vi "Override To Nominal State.vi"(11 "TEMPLATE Queue in":refnum<class "TEMPLATE Queue.lvclass">) -> (3 "TEMPLATE Queue out":refnum<class "TEMPLATE Queue.lvclass">)   [LabVIEW 2021, in "_Template.lvlib" / "Templates.lvlib" / "TEM Queue.lvlib" / "TEMPLATE Queue.lvclass"]
uses:
  TEMPLATE Queue.lvclass
  TEMPLATE Queue.lvclass/TEMPLATE Queue.ctl
  <vilib>/Nathan Davis/jettl/jettl/Queue/Queue.lvclass
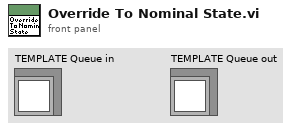
[diagram p1: front panel]
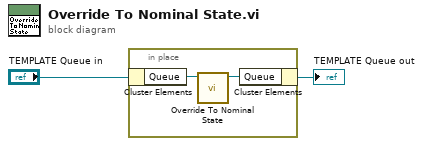
[diagram p0: block diagram]
diagram:
  n1 = in-place {
    n2 = in-place-cluster #1("TEMPLATE Queue in") -> ("Queue"=w4:refnum<class "Queue.lvclass">)
    n3 = call-dynamic "Override To Nominal State.vi"("jettl in"=w4) -> ("jettl out"=w3:refnum<class "Queue.lvclass">)  [unwired: 10 in]
    n4 = in-place-cluster #1("Queue"=w3) -> (→"TEMPLATE Queue out":refnum<class "TEMPLATE Queue.lvclass">)
  }
